vi "3D读取输入.vi"(8 "文件读取路径":path, 9 "时域谱or频域谱":string(combo)="F", 11 "行总数":dbl) -> (0 "文件读取路径":path, 1 "时域谱or频域谱":string(combo), 3 "行总数":dbl)   [LabVIEW 2016]
panel:
  in  "确定":bool
  # "参数输入"
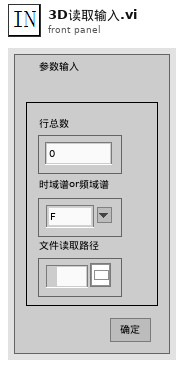
[diagram p1: front panel]
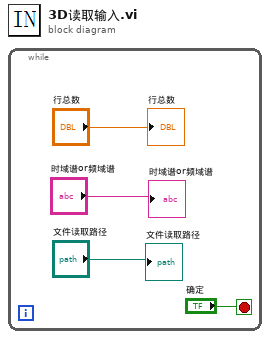
[diagram p0: block diagram]
diagram:
  n1 = while {
    stop <- "确定" stop-if-true
    "行总数" <- "行总数"
    "时域谱or频域谱" <- "时域谱or频域谱"
    "文件读取路径" <- "文件读取路径"
  }
